vi "generateTiffStacks.vi"(1 "singleImgFname":path[][][][](array[path]), 2 "stackFname":path[][][](array[path])) -> (0 "stackGenerationComplete":bool)   [LabVIEW 2015]
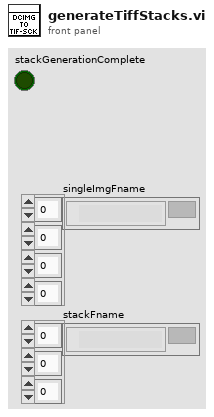
[diagram p1: front panel]
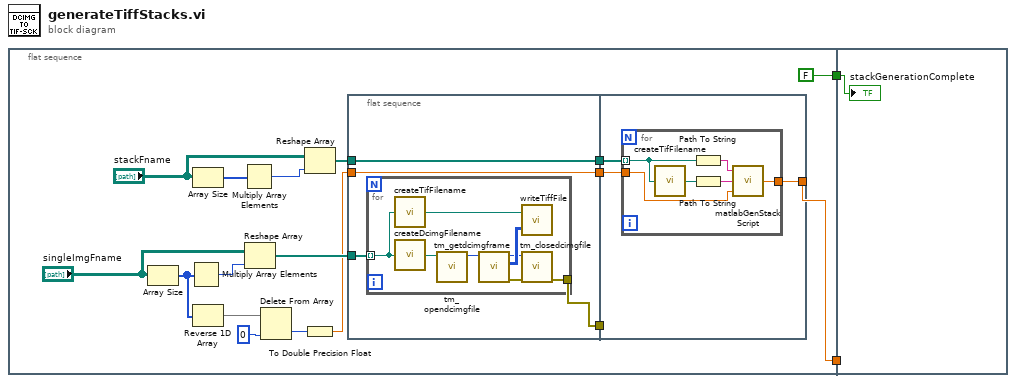
[diagram p0: block diagram]
diagram:
  n1 = flat-sequence {
    tunnel: [FALSE ("stackGenerationComplete")] -> w2
    tunnel: [w8] -> w1
    tunnel: w2 -> [w41]
    tunnel: w1 -> [_]
    frame #0 {
      n2 = Array Size(array="singleImgFname") -> (size(s)=w19:i32[])
      n3 = Multiply Array Elements(1:w19) -> (0:w12:i32)
      n4 = Array Size(array="stackFname") -> (size(s)=w15:i32[])
      n5 = Reverse 1D Array(array=w19) -> (reversed array=w16:i32[])
      n6 = Multiply Array Elements(1:w15) -> (0:w13:i32)
      n7 = Reshape Array("singleImgFname", w12) -> (w14:path[])
      n8 = Delete From Array(array=w16, index=0) -> (deleted portion=w18:i32)  [unwired: 1 in, 1 out]
      n9 = Reshape Array("stackFname", w13) -> (w5:path[])
      n10 = To Double Precision Float(number=w18) -> (double precision float=w6:dbl)
      n11 = flat-sequence {
        tunnel: w14 -> [w23]
        tunnel: [w22] -> w7
        tunnel: w6 -> [w22]
        tunnel: w5 -> [w21]
        tunnel: [w21] -> w4
        tunnel: [w20] -> w3
        tunnel: [w34] -> w8
        tunnel: w7 -> [w33]
        tunnel: w4 -> [w32]
        tunnel: w3 -> [_]
        frame #0 {
          n12 = for {
            tunnel: w23 -> [w31] mode=indexing
            tunnel: [w24] -> w20
            n13 = call "createTifFilename.vi"("inputPath"=w31) -> ("tifPath"=w30:path)
            n14 = call "createDcimgFilename.vi"("origPath"=w31) -> ("dcimgPath"=w29:path)
            n15 = call <userlib>:"tm_opendcimgfile.vi"("Path"=w29) -> ("File Handle"=w27:u32)  [unwired: 8 in, 2 out]
            n16 = call <userlib>:"tm_getdcimgframe.vi"("File Handle in"=w27) -> ("error out"=w26:errorcluster, "Data"=w28:u16[][], "File Handle out"=w25:u32)  [unwired: 7 in, 1 out]
            n17 = call "writeTiffFile.vi"("Image Pixels (U16)"=w28, "File Path"=w30) -> ()
            n18 = call <userlib>:"tm_closedcimgfile.vi"("error in (no error)"=w26, "File Handle"=w25) -> ("error out"=w24:errorcluster)  [unwired: 9 in]
          }
        }
        frame #1 {
          n19 = for {
            tunnel: w32 -> [w39] mode=indexing
            tunnel: w33 -> [w36]
            tunnel: [w35] -> w34
            n20 = call "createTifFilename.vi"("inputPath"=w39) -> ("tifPath"=w40:path)
            n21 = Path To String(path=w39) -> (string=w38:string)
            n22 = Path To String(path=w40) -> (string=w37:string)
            n23 = call "matlabGenStackScript.vi"("noImgsInStack"=w36, "tifStackFname"=w37, "stackFnameBase"=w38) -> ("No stacksGenerated"=w35:dbl)
          }
        }
      }
    }
    frame #1 {
      "stackGenerationComplete" <- w41
    }
  }
